vi "JSON Command.vi"(8 "error in (no error)":errorcluster, 11 "Error Message":string) -> (0 "error out":errorcluster, 3 "JSON string":string)   [LabVIEW 2013, in "Connection Handler.lvlib"]
uses:
  Connection Handler.lvlib
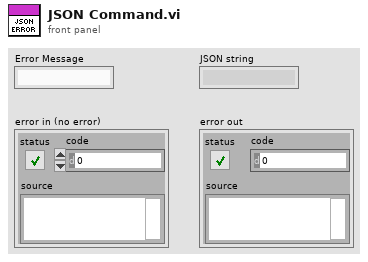
[diagram p1: front panel]
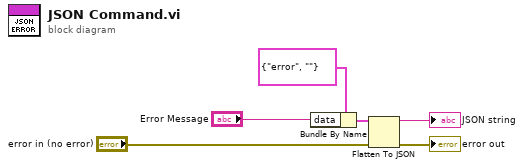
[diagram p0: block diagram]
diagram:
  n1 = Bundle By Name(cluster=cluster{"command":string, "data":string} {"command"="error", "data"=""}, "data"="Error Message") -> (w4:cluster{"command":string, "data":string})
  n2 = Flatten To JSON(anything=w4, error in (no error)="error in (no error)") -> (JSON string=→"JSON string":string, 11:→"error out":errorcluster)  [unwired: 1 in]
